vi "Node HTTP Post.vi"(6 "Timeout ms (10000)":i32=10000, 7 "Node Name":string, 8 "error in (no error)":errorcluster, 9 "Payload":string, 10 "Path":string, 11 "VolatusAPI in":refnum<class "VolatusAPI.lvclass">) -> (0 "error out":errorcluster, 1 "Headers":string, 2 "Response":string, 3 "VolatusAPI out":refnum<class "VolatusAPI.lvclass">, 4 "Status Code":u32)   [LabVIEW 2020, in "Volatus.lvlib" / "VolatusAPI.lvclass"]
uses:
  VolatusAPI.lvclass
  <vilib>/NI/Advanced HTTP Client/Multipart Data--cluster.ctl
  VolatusAPI.lvclass/VolatusAPI.ctl
  <vilib>/NI/Advanced HTTP Client/POST (Multipart).vi
  <vilib>/NI/Advanced HTTP Client/Session.lvclass
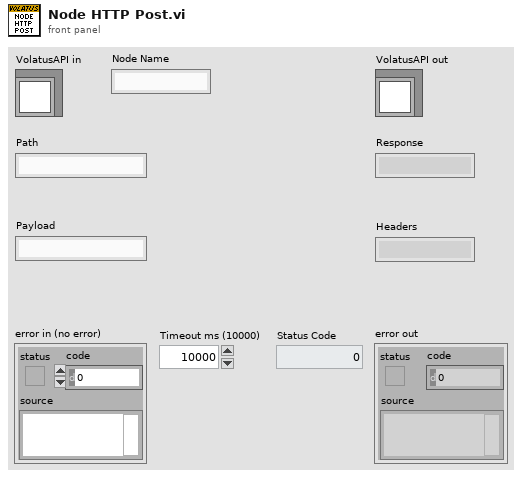
[diagram p1: front panel]
types:
  T1 = typedef "lib_NI_Advanced HTTP Client.lvlib/Session.lvclass/Multipart Data--cluster.ctl" = cluster{"name":string, "value":string, "file":path, "filename":string, "MIME type":string}
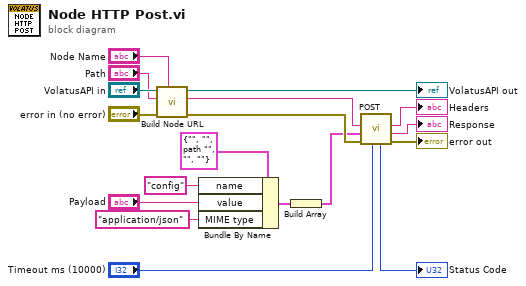
[diagram p0: block diagram]
diagram:
  n1 = call "Build Node URL.vi"("Node Name"="Node Name", "error in (no error)"="error in (no error)", "Path"="Path", "VolatusAPI in"="VolatusAPI in") -> ("error out"=w9:errorcluster, "Request URL"=w10:string, "VolatusAPI out"=→"VolatusAPI out":refnum<class "VolatusAPI.lvclass">)  [unwired: 5 in]
  n2 = Bundle By Name(cluster=T1 {"name"="", "value"="", "file"=path "", "filename"="", "MIME type"=""} ("multipart data"), "name"="config", "value"="Payload", "MIME type"="application/json") -> (w2:T1)
  n3 = Build Array(w2) -> (w1:T1[])
  n4 = call-poly <vilib>:"POST.vi"("timeout"="Timeout ms (10000)", "error in"=w9, "data"=w1, "url"=w10) -> ("error out"=→"error out":errorcluster, "body"=→"Response":string, "headers"=→"Headers":string, "status code"=→"Status Code":u32)  [unwired: 3 in, 1 out]
